vi "only words and commas.vi"(11 "input string":string) -> (3 "result string":string)   [LabVIEW 2019]
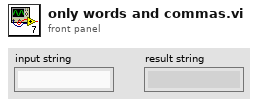
[diagram p1: front panel]
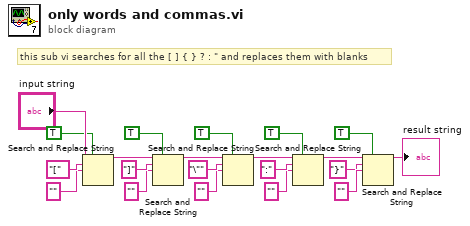
[diagram p0: block diagram]
diagram:
  # "this sub vi searches for all the [ ] { } ? : \" and replaces them with blanks"
  n1 = Search and Replace String(replace all?=TRUE ("replace all? (F)"), input string="input string", search string="[", replace string="" ("replace string (\"\")")) -> (result string=w16:string)  [unwired: 4 in, 3 out]
  n2 = Search and Replace String(replace all?=TRUE ("replace all? (F)"), input string=w16, search string="]", replace string="" ("replace string (\"\")")) -> (result string=w12:string)  [unwired: 4 in, 3 out]
  n3 = Search and Replace String(replace all?=TRUE ("replace all? (F)"), input string=w12, search string="\"", replace string="" ("replace string (\"\")")) -> (result string=w6:string)  [unwired: 4 in, 3 out]
  n4 = Search and Replace String(replace all?=TRUE ("replace all? (F)"), input string=w6, search string=":", replace string="" ("replace string (\"\")")) -> (result string=w2:string)  [unwired: 4 in, 3 out]
  n5 = Search and Replace String(replace all?=TRUE ("replace all? (F)"), input string=w2, search string="}", replace string="" ("replace string (\"\")")) -> (result string=→"result string":string)  [unwired: 4 in, 3 out]
